vi "test_ultrasonic.vi"() -> ()   [LabVIEW 2011]
panel:
  out "Average Distance (in)\nOver 10 readings":dbl
  out "Instantaneous Distance (in)":dbl
  out "Distance Graph (in)":dbl(graph)
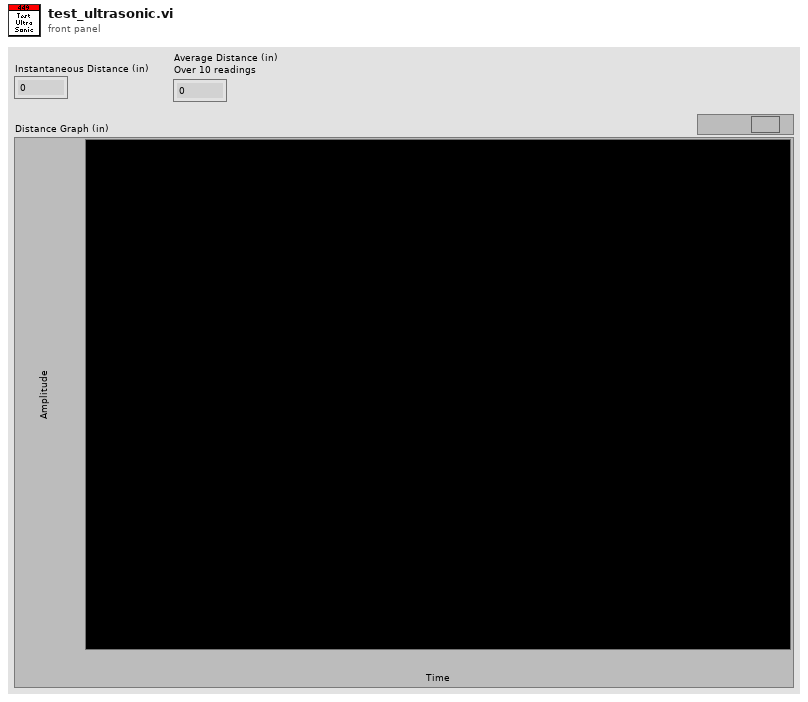
[diagram p1: front panel]
types:
  T1 = typedef "WPI_AnalogChannelDevRef.ctl" = cluster{"DevStatus":errorcluster, "Analog Module":T2, "Analog Channel":T3}
  T2 = typedef "FPGA_TypedefAnalogModule.ctl" = enum16{"Analog Module 1", "Analog Module 2"}
  T3 = typedef "FPGA_AIChannel.ctl" = enum8{"AI 1", "AI 2", "AI 3", "AI 4", "AI 5", "AI 6", "AI 7", "AI 8", "Invalid"}
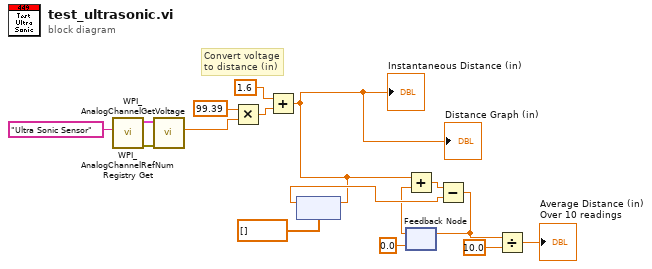
[diagram p0: block diagram]
diagram:
  # "Convert voltage\nto distance (in)"
  n1 = call <vilib>:"WPI_AnalogChannelRefNum Registry Get.vi"("refnum name"="Ultra Sonic Sensor") -> ("error out"=w6:errorcluster, "AIDeviceRef"=w7:T1)  [unwired: 9 in]
  n2 = call <vilib>:"WPI_AnalogChannelGetVoltage.vi"("error in (no error)"=w6, "AIDeviceRef"=w7) -> ("Voltage"=w2:dbl)  [unwired: 7 in, 2 out]
  n3 = Multiply(x=99.39, y=w2) -> (x*y=w4:dbl)
  n4 = Add(x=1.6, y=w4) -> (x+y=w1:dbl)
  "Distance Graph (in)" <- w1
  "Instantaneous Distance (in)" <- w1
  n5 = feedback #1(dbl[] []) -> (w12:dbl)
  n6 = feedback-in #1(w1) -> ()
  n7 = feedback #2(0.0) -> (w10:dbl)
  n8 = Add(x=w1, y=w10) -> (x+y=w11:dbl)
  n9 = Subtract(x=w11, y=w12) -> (x-y=w14:dbl)
  n10 = feedback-in #2(w14) -> ()
  n11 = Divide(x=w14, y=10.0) -> (x/y=→"Average Distance (in)\nOver 10 readings":dbl)
